vi "Trigger Video Query.vi"(0 "Instrument Handle In":i32, 11 "error in":errorcluster) -> (3 "Type":i32, 4 "Instrument Handle Out":i32, 6 "Source":i32, 8 "Level":dbl, 10 "Standard":i32, 13 "Line":i32, 14 "Field":i32, 15 "error out":errorcluster)   [LabVIEW 8.6, in "ZTScopeM.lvlib"]
doc: "Query the video trigger configuration."
uses:
  ZTScopeM.lvlib
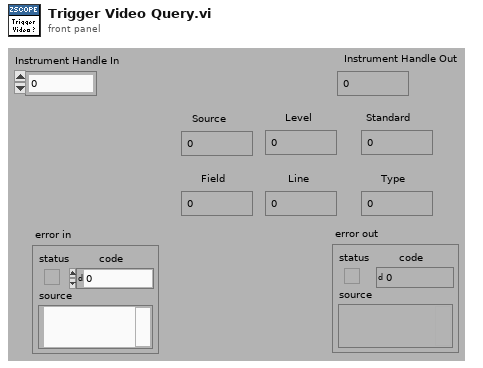
[diagram p1: front panel]
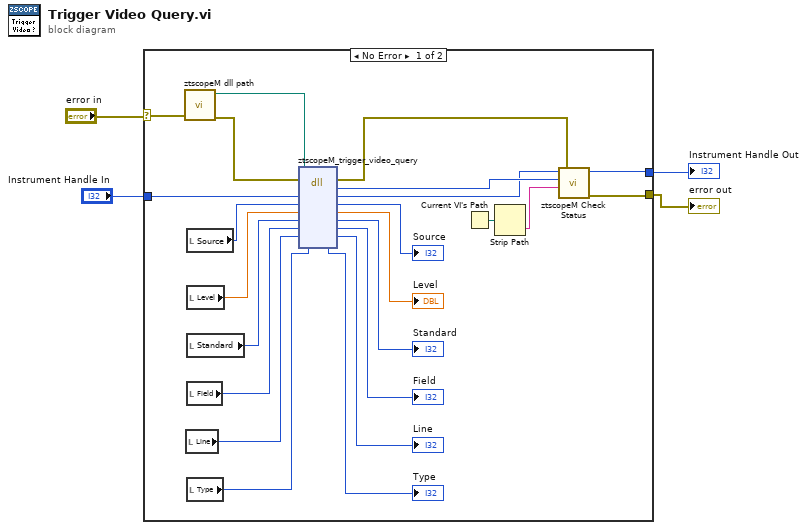
[diagram p0: block diagram]
diagram:
  n1 = case shown="No Error" "error in" {
    selector: "error in" -> [w8 w29]
    tunnel: [w9 w29] -> w1
    tunnel: "Instrument Handle In" -> [w27 w28]
    tunnel: [w10 w28] -> w3
    frame #0 {
      n2 = call "ztscopeM dll path.vi"("error in (no error)"=w8) -> ("error out"=w6:errorcluster, "<instrument>.dll path"=w7:path)  [unwired: 9 in]
      n3 = local read "Line"() -> (w18:i32)
      n4 = local read "Source"() -> (w26:i32)
      n5 = local read "Level"() -> (w24:dbl)
      n6 = local read "Standard"() -> (w22:i32)
      n7 = local read "Field"() -> (w20:i32)
      n8 = local read "Type"() -> (w16:i32)
      n9 = dll-call lib="C:/Program Files (x86)/National Instruments/LabVIEW 2013/instr.lib/ztscopem/ztscopeM.dll" fn="ztscopeM_trigger_video_query"(path in=w7, error in=w6, "instrumentHandle"=w27, "source"=w26, "level"=w24, "standard"=w22, "field"=w20, "line"=w18, "type"=w16) -> (error out=w5:errorcluster, w12:i32, "instrumentHandle"=w11:i32, "source"=→"Source":i32, "level"=→"Level":dbl, "standard"=→"Standard":i32, "field"=→"Field":i32, "line"=→"Line":i32, "type"=→"Type":i32)  [unwired: 1 in, 1 out]
      n10 = Current VI's Path() -> (path=w14:path)
      n11 = Strip Path(path=w14) -> (name=w13:string)  [unwired: 1 out]
      n12 = call "ztscopeM Check Status.vi"("error in"=w5, "name of VI"=w13, "status (return code)"=w12, "instrument handle in"=w11) -> ("error out"=w9:errorcluster, "instrument handle out"=w10:i32)  [unwired: 2 in]
    }
    frame #1 {
    }
  }
  "Instrument Handle Out" <- w3
  "error out" <- w1
